vi "구조공부.vi"() -> ()   [LabVIEW 2018]
uses:
  <vilib>/Utility/tcp.llb/UDP Multicast Read-Only Open.vi
  auto_update_server/Module/Message Queue/Enqueue Message (Single).vi
  auto_update_server/Module/Message Queue/Message Queue.lvlib
panel:
  out "ccc":bool
  out "bbb":bool
  out "aaa":bool
  out "데이터 출력":string
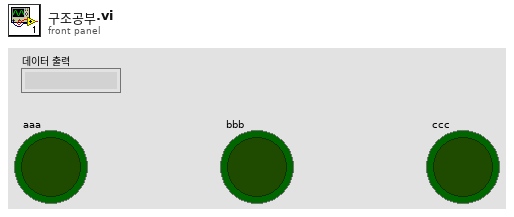
[diagram p1: front panel]
types:
  T1 = typedef "Message Queue.lvlib/All Message Queues.ctl" = cluster{"UI":refnum<queue>, "Display":refnum<queue>, "Timer":refnum<queue>}
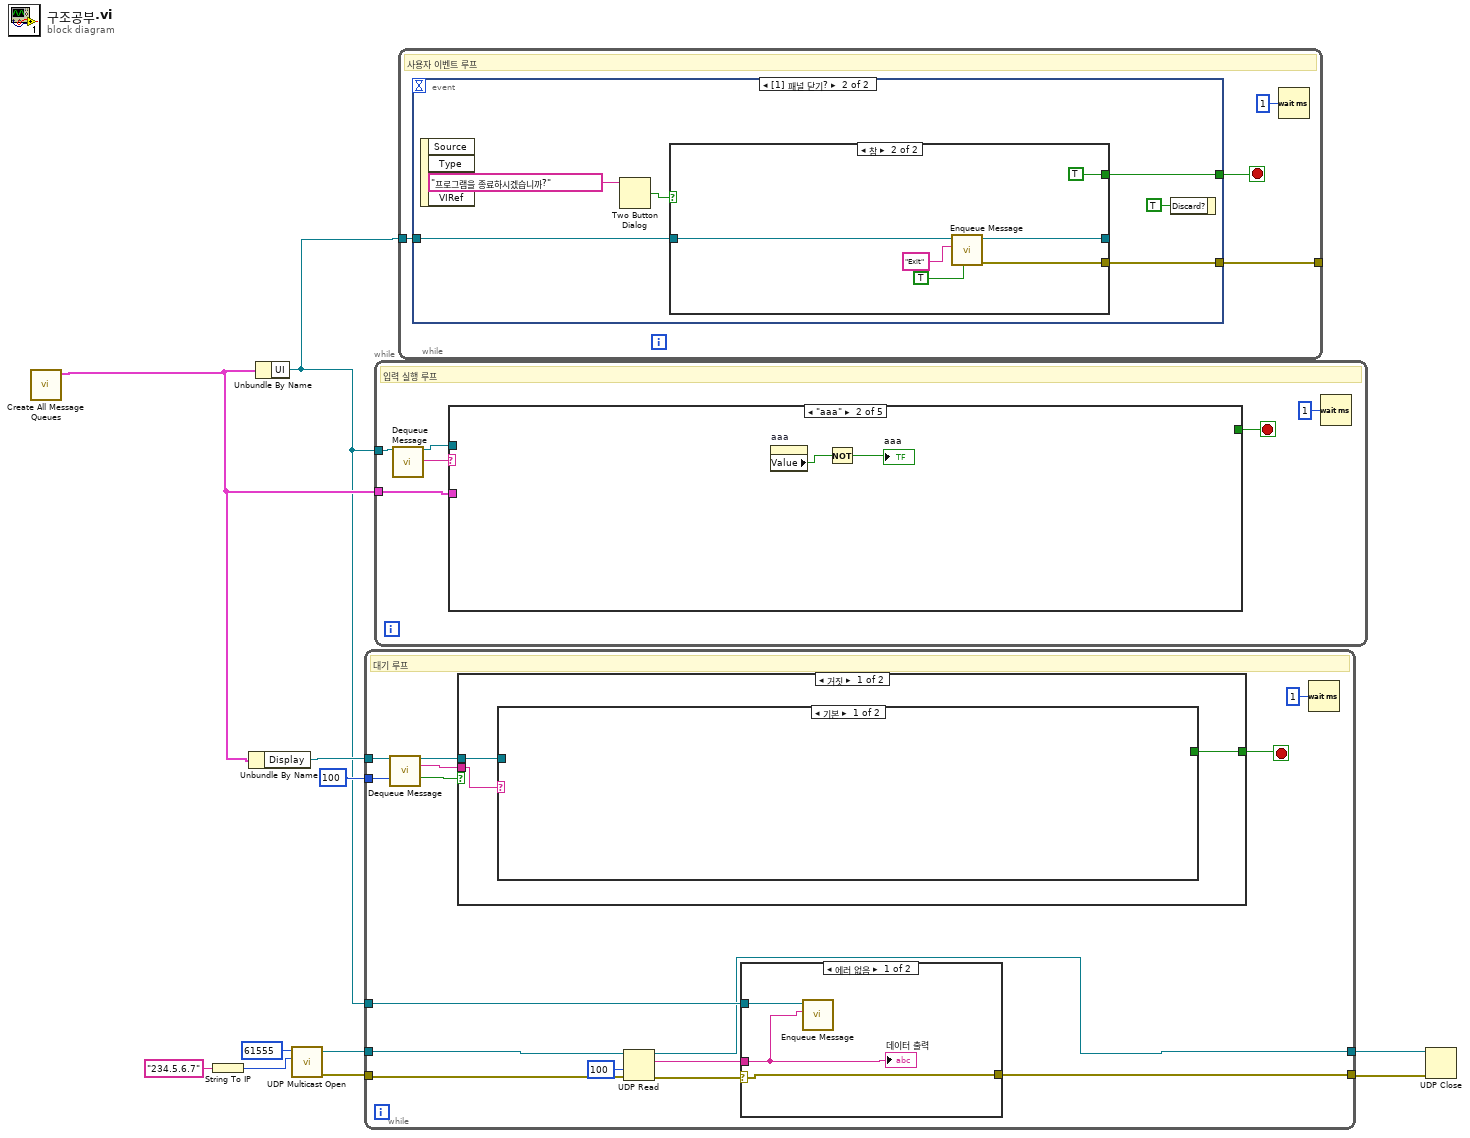
[diagram p0: block diagram]
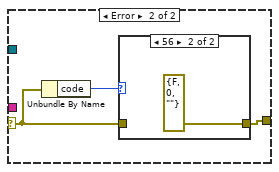
[diagram p2: hidden frame]
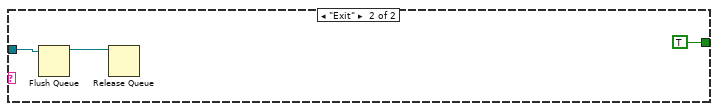
[diagram p4: hidden frame]
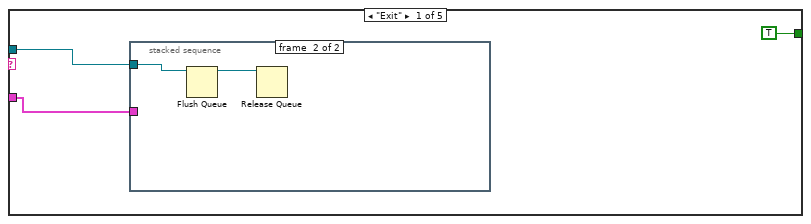
[diagram p6: hidden frame]
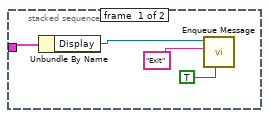
[diagram p7: hidden frame]
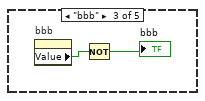
[diagram p8: hidden frame]
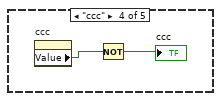
[diagram p9: hidden frame]
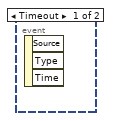
[diagram p11: hidden frame]
diagram:
  n1 = call "Create All Message Queues.vi"() -> ("Message Queues out"=w9:T1)  [unwired: 10 in, 1 out]
  n2 = String To IP(1:"234.5.6.7" ("이름")) -> (0:w6:u32)
  n3 = Unbundle By Name(w9) -> ("Display"=w11:refnum<queue>)
  n4 = Unbundle By Name(w9) -> ("UI"=w3:refnum<queue>)
  n5 = call-poly <vilib>:"UDP Multicast Open.vi"("multicast addr"=w6, "port"=u16 61555 ("포트")) -> ("error out"=w4:errorcluster, "connection ID"=w5:refnum<k16>)  [unwired: 7 in, 1 out]
  n6 = while {
    tunnel: w11 -> [w26]
    tunnel: 100 ("타임아웃(ms) (-1)") -> [w25]
    tunnel: w5 -> [w20]
    tunnel: w4 -> [w19]
    tunnel: w3 -> [w18]
    tunnel: [w17] -> w2
    tunnel: [w16] -> w1
    stop <- w21 stop-if-true
    # "대기 루프"
    n7 = call "Dequeue Message.vi"("Message Queue"=w26, "타임아웃(ms) (-1)"=w25) -> ("dup Message Queue"=w22:refnum<queue>, "Message"=w23:string, "타임아웃?"=w24:bool)  [unwired: 9 in, 2 out]
    n8 = case shown="거짓" w24 {
      tunnel: w23 -> [w37 _]
      tunnel: w22 -> [w36 _]
      tunnel: [w35 _] -> w21
      frame False {
        n9 = case shown="기본" w37 {
          tunnel: w36 -> [_ w39]
          tunnel: [_ TRUE] -> w35
          frame Default {
          }
          frame "Exit" {
            n10 = Flush Queue(queue=w39) -> (queue out=w40:refnum<queue>)  [unwired: 1 in, 2 out]
            n11 = Release Queue(queue=w40) -> ()  [unwired: 2 in, 3 out]
          }
        }
      }
      frame True {
      }
    }
    n12 = UDP Read(connection ID=w20, timeout ms (25000)=100 ("타임아웃 ms (25000)"), 8:w19) -> (data out=w14:string, error out=w15:errorcluster, 3:w17:refnum<k16>)  [unwired: 1 in, 2 out]
    n13 = case shown="에러 없음" w15 {
      selector: w15 -> [w29 w30]
      tunnel: [w29 w31] -> w16
      tunnel: w14 -> [w28 _]
      tunnel: w18 -> [w27 _]
      frame No Error {
        n14 = call-poly "Enqueue Message.vi"("Message"=w28, "Message Queue"=w27) -> ()  [unwired: 8 in, 2 out]
        "데이터 출력" <- w28
      }
      frame Error {
        n15 = Unbundle By Name(w30) -> ("code"=w32:i32)
        n16 = case shown="56" w32 {
          tunnel: [w33 errorcluster {"status"=FALSE, "code"=0, "source"=""} ("에러 상수")] -> w31
          tunnel: w30 -> [w33 _]
          frame Default {
          }
          frame 56 {
          }
        }
      }
    }
    n17 = Wait (ms)(milliseconds to wait=u32 1 ("대기 시간 (ms)")) -> ()  [unwired: 1 out]
  }
  n18 = while {
    tunnel: w3 -> [w46]
    tunnel: w9 -> [w44]
    stop <- w42 stop-if-true
    # "입력 실행 루프"
    n19 = call "Dequeue Message.vi"("Message Queue"=w46) -> ("dup Message Queue"=w43:refnum<queue>, "Message"=w45:string)  [unwired: 10 in, 3 out]
    n20 = case shown="\"aaa\"" w45 {
      tunnel: w44 -> [w49 _ _ _ _]
      tunnel: w43 -> [w48 _ _ _ _]
      tunnel: [TRUE _ _ _ _] -> w42
      frame "Exit" {
        n21 = stacked-sequence {
          tunnel: w49 -> [w53 _]
          tunnel: w48 -> [_ w55]
          frame #0 {
            n22 = Unbundle By Name(w53) -> ("Display"=w52:refnum<queue>)
            n23 = call-poly "Enqueue Message.vi"("Priority Message? (F)"=TRUE, "Message"="Exit", "Message Queue"=w52) -> ()  [unwired: 7 in, 2 out]
          }
          frame #1 {
            n24 = Flush Queue(queue=w55) -> (queue out=w54:refnum<queue>)  [unwired: 1 in, 2 out]
            n25 = Release Queue(queue=w54) -> ()  [unwired: 2 in, 3 out]
          }
        }
      }
      frame "aaa" {
        n26 = property on="aaa" class="Bool (엄격한)"() -> ("Value"=w57:bool)  [unwired: 2 in, 2 out]
        n27 = Not(x=w57) -> (.not. x?=→"aaa":bool)
      }
      frame "bbb" {
        n28 = property on="bbb" class="Bool (엄격한)"() -> ("Value"=w59:bool)  [unwired: 2 in, 2 out]
        n29 = Not(x=w59) -> (.not. x?=→"bbb":bool)
      }
      frame "ccc" {
        n30 = property on="ccc" class="Bool (엄격한)"() -> ("Value"=w61:bool)  [unwired: 2 in, 2 out]
        n31 = Not(x=w61) -> (.not. x?=→"ccc":bool)
      }
      frame Default {
      }
    }
    n32 = Wait (ms)(milliseconds to wait=u32 1 ("대기 시간 (ms)")) -> ()  [unwired: 1 out]
  }
  n33 = while "While 루프" {
    tunnel: [w65] -> _
    tunnel: w3 -> [w64]
    stop <- w63 stop-if-true
    # "사용자 이벤트 루프"
    n34 = event shown="[1] 패널 닫기?" {
      selector: _ -> [_ _]
      dyn-events: _ -> [_ _]
      timeout: _ -> [_ _]
      tunnel: [_ w68] -> w65
      tunnel: w64 -> [_ w67]
      tunnel: [_ w66] -> w63
      event Timeout {
        n35 = event-data() -> ()  [unwired: 1 in, 3 out]
      }
      event Panel Close? {
        n36 = event-data() -> ()  [unwired: 1 in, 4 out]
        n37 = Two Button Dialog(message="프로그램을 종료하시겠습니까?" ("메시지")) -> (T button?=w69:bool)  [unwired: 2 in]
        n38 = case shown="참" w69 {
          tunnel: [_ w76] -> w68
          tunnel: [_ TRUE] -> w66
          tunnel: w67 -> [w72 w74]
          tunnel: [w72 w73] -> _
          frame False {
          }
          frame True {
            n39 = call-poly "Enqueue Message.vi"("Priority Message? (F)"=TRUE, "Message"="Exit", "Message Queue"=w74) -> ("error out"=w76:errorcluster, "dup Message Queue"=w73:refnum<queue>)  [unwired: 7 in]
          }
        }
        n40 = event-data("Discard?"=TRUE ("버림?")) -> ()  [unwired: 1 in, 1 out]
      }
    }
    n41 = Wait (ms)(milliseconds to wait=u32 1 ("대기 시간 (ms)")) -> ()  [unwired: 1 out]
  }
  n42 = UDP Close(connection ID=w2, 8:w1) -> ()  [unwired: 2 out]
